vi "write_params.vi"(8 "error in (no error)":errorcluster, 10 "params":T1={"n_nonzero_coefs"={"n_nonzero_coefs_type"="None", "n_nonzero_coefs_int"=0.0}, "tol"={"tol_type"="None", "tol_float"=0.0}, "fit_intercept"=TRUE, "normalize"=TRUE, "precompute"={"precompute_type"="auto", "precompute_bool"=FALSE}}, 11 "OrthogonalMatchingPursuit in":refnum<class "OrthogonalMatchingPursuit.lvclass">) -> (0 "error out":errorcluster, 3 "OrthogonalMatchingPursuit out":refnum<class "OrthogonalMatchingPursuit.lvclass">)   [LabVIEW 2020, in "OrthogonalMatchingPursuit.lvclass"]
uses:
  OrthogonalMatchingPursuit.lvclass
  Controls/orthogonal_matching_pursuit_params.ctl
  OrthogonalMatchingPursuit.lvclass/OrthogonalMatchingPursuit.ctl
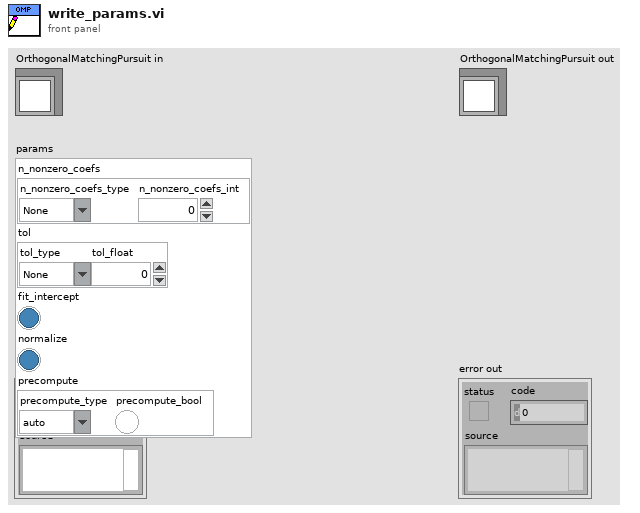
[diagram p1: front panel]
types:
  T1 = typedef "orthogonal_matching_pursuit_params.ctl" = cluster{"n_nonzero_coefs":cluster{"n_nonzero_coefs_type":string, "n_nonzero_coefs_int":dbl}, "tol":cluster{"tol_type":string, "tol_float":dbl}, "fit_intercept":bool, "normalize":bool, "precompute":cluster{"precompute_type":string, "precompute_bool":bool}}
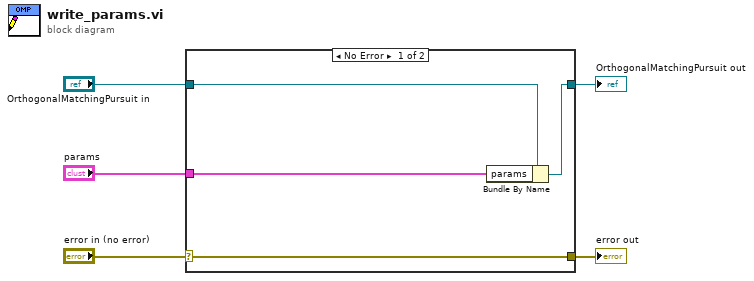
[diagram p0: block diagram]
diagram:
  n1 = case shown="No Error" "error in (no error)" {
    selector: "error in (no error)" -> [w9 w10]
    tunnel: [w9 w10] -> w4
    tunnel: [w7 w11] -> w2
    tunnel: "OrthogonalMatchingPursuit in" -> [w8 w11]
    tunnel: "params" -> [w6 _]
    frame No Error {
      n2 = Bundle By Name(cluster=w8, "params"=w6) -> (w7:refnum<class "OrthogonalMatchingPursuit.lvclass">)
    }
    frame Error {
    }
  }
  "error out" <- w4
  "OrthogonalMatchingPursuit out" <- w2
